vi "Termometr.vi"() -> ()   [LabVIEW 2023]
uses:
  <vilib>/numeric/Random Number (Range) U64.vi
  <vilib>/numeric/sub_Random U32.vi
panel:
  in  "stop":bool
  in  "Skala temperatury":bool
  out "Temperatura [F]":dbl(slide) scale=0.0..100.0
  out "Temperatura [C]":dbl(slide) scale=0.0..100.0 scale format="%#_6f"
  # "deg C"
  # "def F"
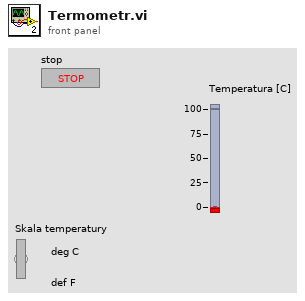
[diagram p1: front panel]
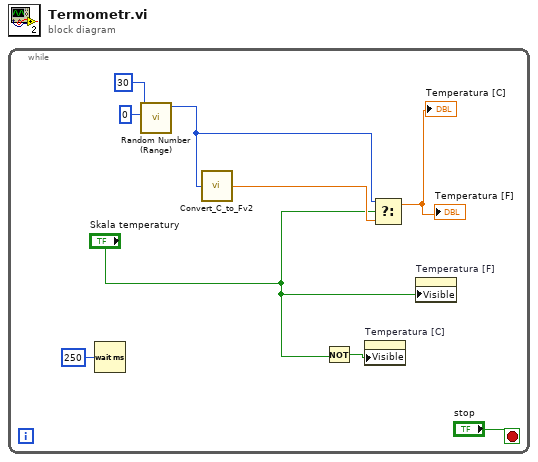
[diagram p0: block diagram]
diagram:
  n1 = while {
    stop <- "stop" stop-if-true
    n2 = Wait (ms)(milliseconds to wait=u32 250) -> ()  [unwired: 1 out]
    n3 = call-poly <vilib>:"Random Number (Range).vi"("lower bound (0)"=u64 0, "upper bound (100)"=u64 30) -> ("number"=w7:u64)  [unwired: 9 in]
    n4 = call "Convert_C_to_Fv2.vi"("deg C"=w7) -> ("deg F"=w5:dbl)
    n5 = Not(x="Skala temperatury") -> (.not. x?=w4:bool)
    n6 = property on="Temperatura [C]" class="Slide (strict)"("Visible"=w4) -> ()  [unwired: 2 in, 2 out]
    n7 = Select(t=w7, s="Skala temperatury", f=w5) -> (s? t:f=→"Temperatura [C]" →"Temperatura [F]":dbl)
    n8 = property on="Temperatura [F]" class="Slide (strict)"("Visible"="Skala temperatury") -> ()  [unwired: 2 in, 2 out]
  }
